vi "run.create_free.vi"(8 "error in":errorcluster, 11 "RunCreateStaging":refnum<class "RunCreateStaging.lvclass">) -> (0 "error out":errorcluster)   [LabVIEW 2020, in "RunCreateStaging.lvclass"]
doc: "Releases the handle and its associated resources."
uses:
  RunCreateStaging.lvclass
  RunCreateStaging.lvclass/RunCreateStaging.ctl
  client.lvlib
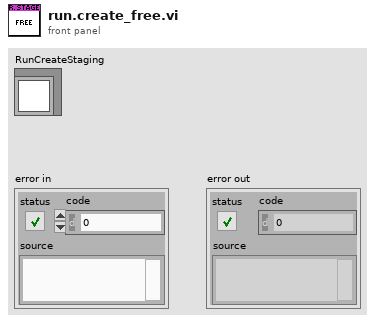
[diagram p1: front panel]
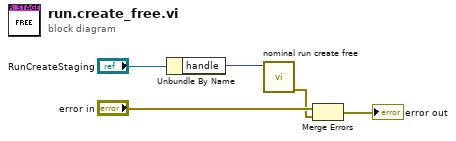
[diagram p0: block diagram]
diagram:
  n1 = Unbundle By Name("RunCreateStaging") -> ("handle"=w5:i32)
  n2 = call "nominal run create free.vi"("staging"=w5) -> ("error out"=w2:errorcluster)  [unwired: 9 in, 1 out]
  n3 = Merge Errors("error in", w2) -> (→"error out":errorcluster)
